vi "Find Macro String Constant from Frame.vi"(8 "error in (no error)":errorcluster, 11 "Diagram in":refnum<vi>) -> (0 "error out":errorcluster, 1 "Found?":bool, 2 "Macro String Constant":refnum<vi>, 4 "All String Constants":refnum<vi>[](array[refnum]))   [LabVIEW 2013, in "JKI State Machine API.lvlib" / "JKI SM.lvclass"]
uses:
  JKI SM.lvclass
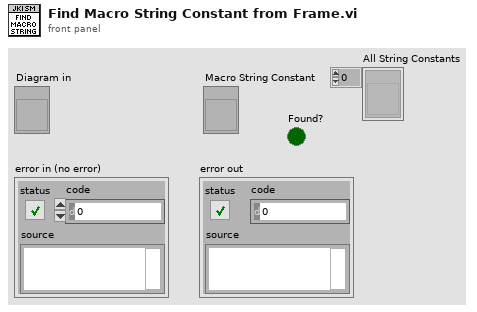
[diagram p1: front panel]
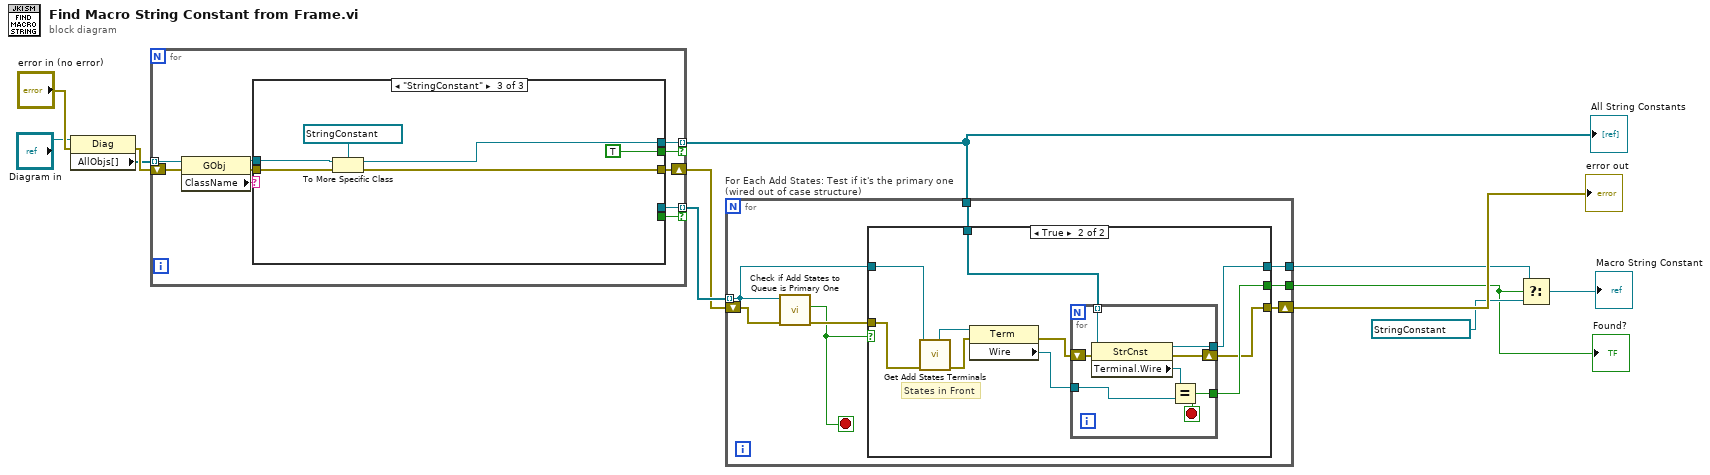
[diagram p0: block diagram]
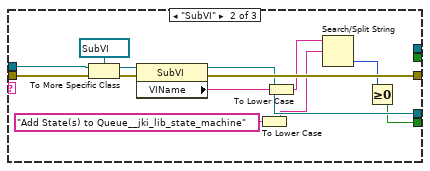
[diagram p4: hidden frame]
diagram:
  n1 = property class="Diag"(reference="Diagram in", error in="error in (no error)") -> (error out=w11:errorcluster, "AllObjs[]"=w10:refnum<vi>[])  [unwired: 1 out]
  n2 = for {
    tunnel: w10 -> [w19] mode=indexing
    shift-right: [w18] -> w7
    shift-left: w11 -> [w17]
    tunnel: [w16] -> w8 mode=indexing if=w15
    tunnel: [w14] -> w5 mode=indexing if=w13
    n3 = property class="GObj"(reference=w19, error in=w17) -> (reference out=w21:refnum<vi>, error out=w20:errorcluster, "ClassName"=w22:string)
    n4 = case shown="\"StringConstant\"" w22 {
      tunnel: w21 -> [_ w35 w42]
      tunnel: w20 -> [w23 w34 w41]
      tunnel: [w23 w29 w40] -> w18
      tunnel: [_ w28 _] -> w16
      tunnel: [_ w27 _] -> w15
      tunnel: [_ _ w38] -> w14
      tunnel: [_ _ TRUE] -> w13
      frame Default {
      }
      frame "SubVI" {
        n5 = To More Specific Class(target class=refnum<vi> refnum ("SubVI Refnum"), reference=w35, error in=w34) -> (specific class reference=w33:refnum<vi>, error out=w32:errorcluster)
        n6 = property class="SubVI"(reference=w33, error in=w32) -> (reference out=w28:refnum<vi>, error out=w29:errorcluster, "VIName"=w31:string)
        n7 = To Lower Case(string="Add State(s) to Queue__jki_lib_state_machine" ("VI Name")) -> (all lower case string=w25:string)
        n8 = To Lower Case(string=w31) -> (all lower case string=w26:string)
        n9 = Search/Split String(string=w26, search string/char (-)=w25) -> (offset of match=w24:i32)  [unwired: 1 in, 2 out]
        n10 = Greater Or Equal To 0?(x=w24) -> (x >= 0?=w27:bool)
      }
      frame "StringConstant" {
        n11 = To More Specific Class(target class=refnum<vi> refnum ("StrCnst Refnum"), reference=w42, error in=w41) -> (specific class reference=w38:refnum<vi>, error out=w40:errorcluster)
      }
    }
  }
  "All String Constants" <- w5
  n12 = for "For Each Add States: Test if it's the primary one (wired out of case structure)" {
    tunnel: w8 -> [w49] mode=indexing
    shift-right: [w43] -> w6
    shift-left: w7 -> [w50]
    tunnel: w5 -> [w47]
    tunnel: [w46] -> w4
    tunnel: [w44] -> w1
    stop <- w45 stop-if-true
    n13 = call "Check if Add States to Queue is Primary One.vi"("error in (no error)"=w50, "Add State(s) to Queue ref"=w49) -> ("error out"=w48:errorcluster, "Is Primary?"=w45:bool)  [unwired: 8 in]
    n14 = case shown="True" w45 {
      tunnel: w49 -> [_ w61]
      tunnel: w48 -> [w51 w59]
      tunnel: w47 -> [_ w58]
      tunnel: [_ w56] -> w46
      tunnel: [_ w55] -> w44
      tunnel: [w51 w52] -> w43
      frame False {
      }
      frame True {
        # "States in Front"
        n15 = call "Get Add States Terminals.vi"("error in (no error)"=w59, "Add State(s) to Queue ref"=w61) -> ("error out"=w54:errorcluster, "State(s) in Front (\"\")"=w60:refnum<vi>)  [unwired: 5 in, 3 out]
        n16 = property class="Term"(reference=w60, error in=w54) -> (error out=w53:errorcluster, "Wire"=w57:refnum<vi>)  [unwired: 1 out]
        n17 = for {
          tunnel: w58 -> [w68] mode=indexing
          tunnel: w57 -> [w66]
          tunnel: [w65] -> w56
          tunnel: [w64] -> w55
          shift-right: [w62] -> w52
          shift-left: w53 -> [w63]
          stop <- w64 stop-if-true
          n18 = property class="StrCnst"(reference=w68, error in=w63) -> (reference out=w65:refnum<vi>, error out=w62:errorcluster, "Terminal.Wire"=w67:refnum<vi>)
          n19 = Equal?(x=w67, y=w66) -> (x = y?=w64:bool)
        }
      }
    }
  }
  "error out" <- w6
  "Found?" <- w1
  n20 = Select(t=w4, s=w1, f=refnum<vi> refnum) -> (s? t:f=→"Macro String Constant":refnum<vi>)
